vi "TestRubyFit.vi"() -> ()   [LabVIEW 2016]
uses:
  Multi-peak Parameters.ctl
  Peak Parameters.ctl
panel:
  in  "File Path Control":path
  in  "Fit parameters":T1={"Peaks"=[{"Amplitude"=10000.0, "Center"=694.3, "Width"=0.8}, {"Amplitude"=8000.0, "Center"=692.0, "Width"=0.6}], "Slope"=0.0, "Intercept"=1500.0, "Function"=enum."Lorentz"}
  in  "Use last fit as  guess":bool
  in  "Reference wavelengh":dbl=694.123
  out "Pressure, kBar":dbl=7.520465813546207 format="%#_4g"
  out "Fit result":T1={"Peaks"=[{"Amplitude"=760.8878418864276, "Center"=694.3954806454184, "Width"=1e-07}, {"Amplitude"=264.42405026147753, "Center"=691.2120066899422, "Width"=1e-07}], "Slope"=-1.0993239942180182, "Intercept"=1795.7475609605895, "Function"=enum."Lorentz"}
  in  "Repeat":i32=3
  in  "Window end":dbl=697.0
  in  "Window start":dbl=690.0
  out "Spectral Waveform":T3(graph)
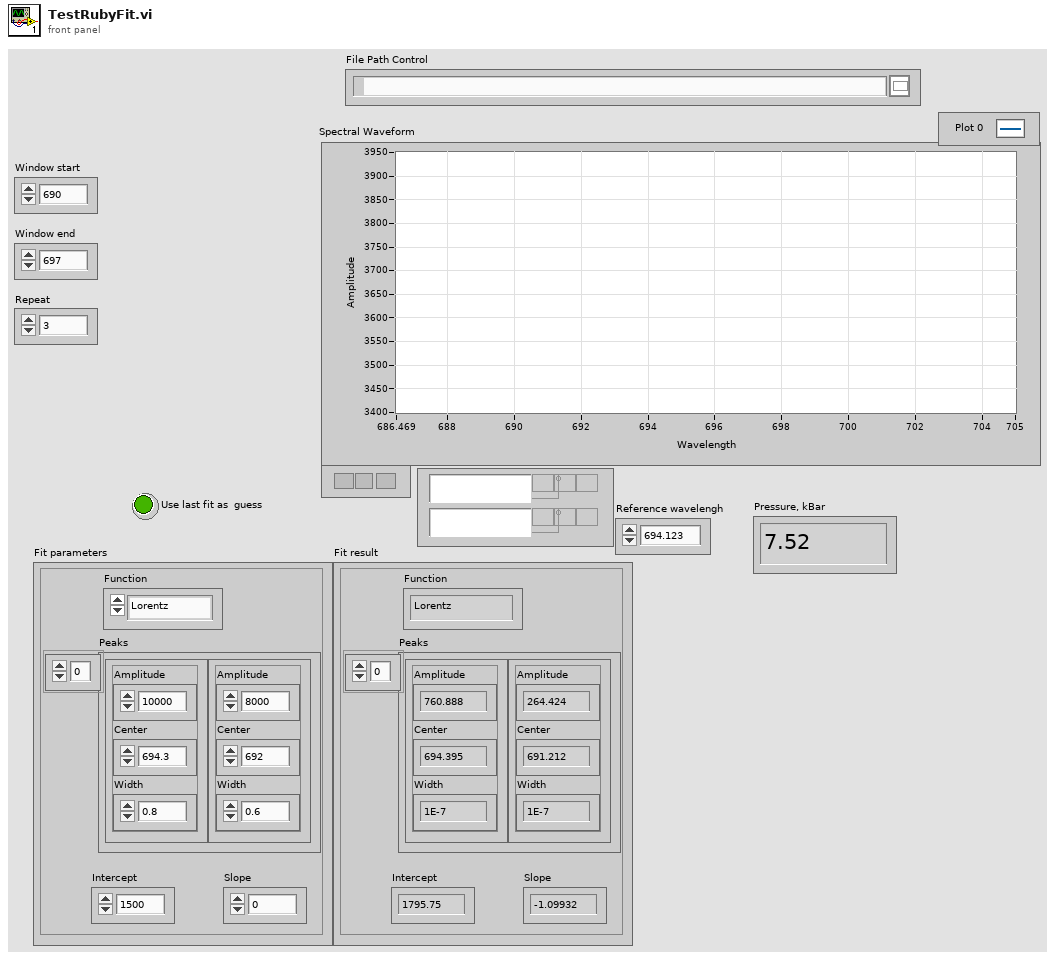
[diagram p1: front panel]
types:
  T1 = typedef "Multi-peak Parameters.ctl" = cluster{"Peaks":T2[], "Slope":dbl, "Intercept":dbl, "Function":enum16{"Gauss", "Lorentz"}}
  T2 = typedef "Peak Parameters.ctl" = cluster{"Amplitude":dbl, "Center":dbl, "Width":dbl}
  T3 = cluster{"Wavelength (nm)":dbl[], "Spectrum by Pixel Number":dbl[]}[]
  T4 = enum16{"open", "open or create", "create or replace", "create", "open (read-only)"}
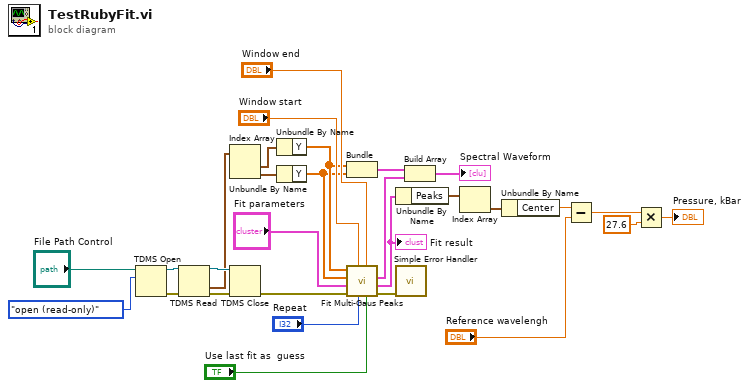
[diagram p0: block diagram]
diagram:
  n1 = TDMS Open(10:T4."open (read-only)" ("operation (0:open)"), 11:"File Path Control") -> (0:w11:errorcluster, 3:w12:refnum<k34>)  [unwired: 5 in]
  n2 = TDMS Read(0:w12, 11:w11) -> (4:w10:refnum<k34>, 10:w6:waveform(dbl)[], 15:w9:errorcluster)  [unwired: 6 in, 3 out]
  n3 = Index Array(array=w6) -> (element #1=w5:waveform(dbl), element #2=w4:waveform(dbl))  [unwired: 2 in]
  n4 = TDMS Close(8:w9, 11:w10) -> (0:w8:errorcluster)  [unwired: 1 out]
  n5 = Unbundle By Name(w5) -> ("Y"=w2:dbl[])
  n6 = Unbundle By Name(w4) -> ("Y"=w1:dbl[])
  n7 = Bundle("Y"=w2, "Y"=w1) -> (w3:cluster{"Y":dbl[], "Y":dbl[]})  [unwired: 1 out]
  n8 = call "Fit Multi-Gaus Peaks.vi"("Use last fit as  guess"="Use last fit as  guess", "Window end"="Window end", "Repeat"="Repeat", "Window start"="Window start", "Error In"=w8, "Fit parameters"="Fit parameters", "Y"=w1, "X"=w2) -> ("Error Out"=w29:errorcluster, "Fit parameters out"=w24:T1, "Fit plot"=w17:cluster{"Array":dbl[], "Array":dbl[]})  [unwired: 1 in]
  "Fit result" <- w24
  n9 = Unbundle By Name(w24) -> ("Peaks"=w15:T2[])
  n10 = call <vilib>:"Simple Error Handler.vi"("error in (no error)"=w29) -> ()  [unwired: 1 in, 8 out]
  n11 = Build Array(w3, w17) -> (→"Spectral Waveform":cluster{"Array":dbl[], "Array":dbl[]}[])
  n12 = Index Array(array=w15) -> (element=w23:T2)  [unwired: 1 in]
  n13 = Unbundle By Name(w23) -> ("Center"=w22:dbl)
  n14 = Subtract(x=w22, y="Reference wavelengh") -> (x-y=w20:dbl)
  n15 = Multiply(x=w20, y=27.6) -> (x*y=→"Pressure, kBar":dbl)
